vi "Auto2-CubeSwitch.vi"(5 "End By Time":timestamp, 7 "Start Time":timestamp, 11 "Game Data":string) -> (3 "Actual End Time":timestamp)   [LabVIEW 2017]
uses:
  AutoSubsystem/AutoInput.ctl
  AutoSubsystem/AutoSubroutine.lvclass
  DriveAutoData.ctl
  AutoSubsystem/AutoDrive/AutoDrive.lvclass
  AutoSubsystem/AutoOutput.ctl
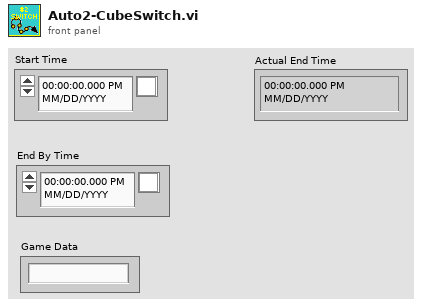
[diagram p1: front panel]
types:
  T1 = typedef "AutoSubroutine.lvclass/AutoInput.ctl" = cluster{"Start by (s)":dbl, "End by (s)":dbl, "Auto Start Time":timestamp, "Local Start":timestamp, "Okay To Start":bool, "End By Time":timestamp}
  T2 = typedef "AutoDrive.lvclass/DriveAutoData.ctl" = cluster{"LinearControlMethod":enum16{"Feedback", "Time"}, "Initial gyro angle":dbl}
  T3 = typedef "AutoSubroutine.lvclass/AutoOutput.ctl" = cluster{"Ended Safe?":bool, "True Start (s)":dbl, "True End (s)":dbl}
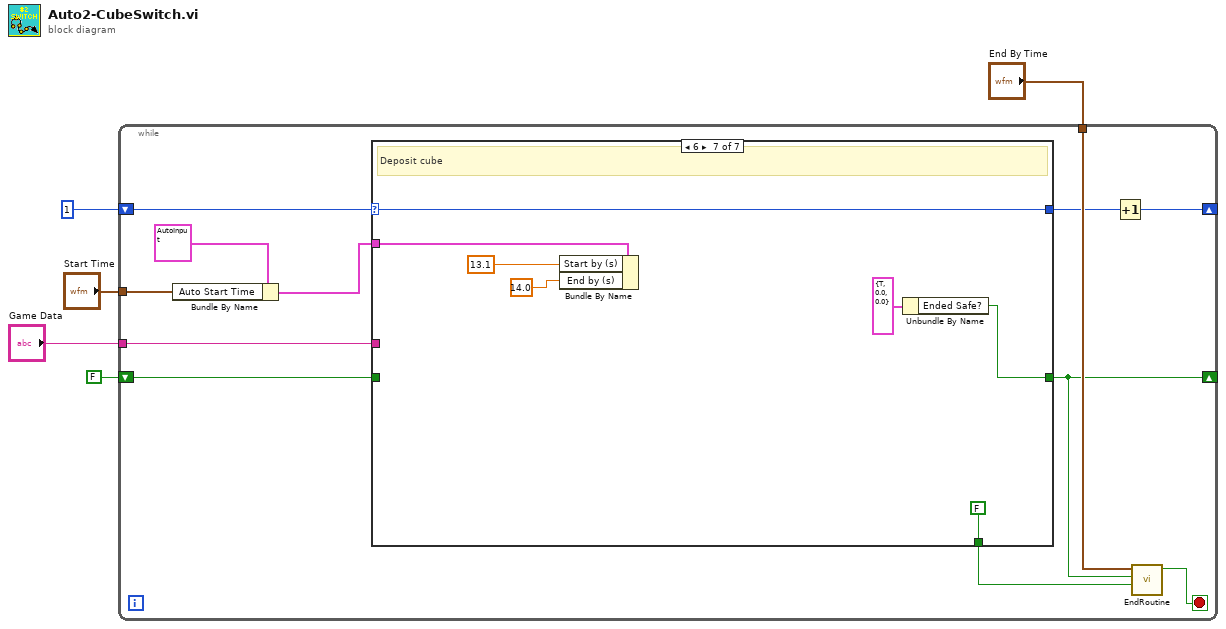
[diagram p0: block diagram]
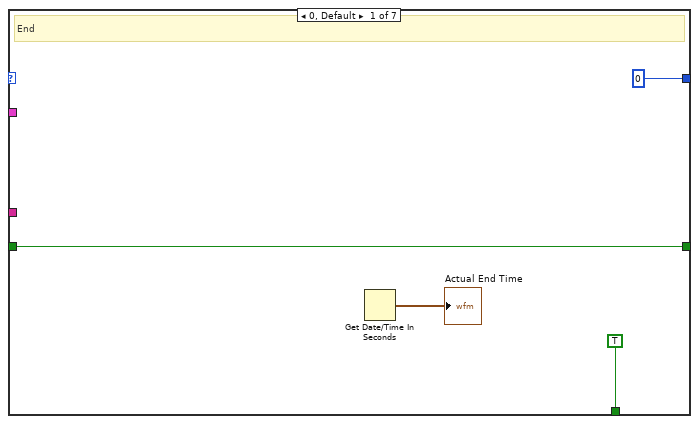
[diagram p2: hidden frame]
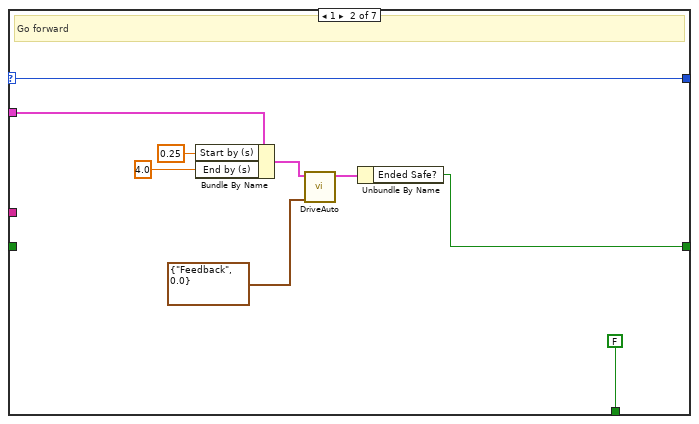
[diagram p3: hidden frame]
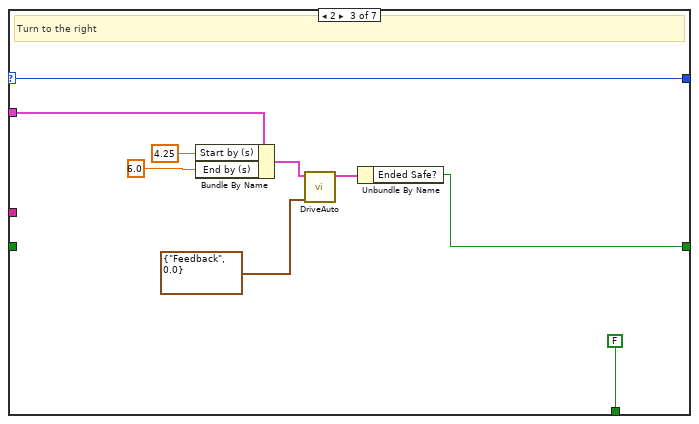
[diagram p4: hidden frame]
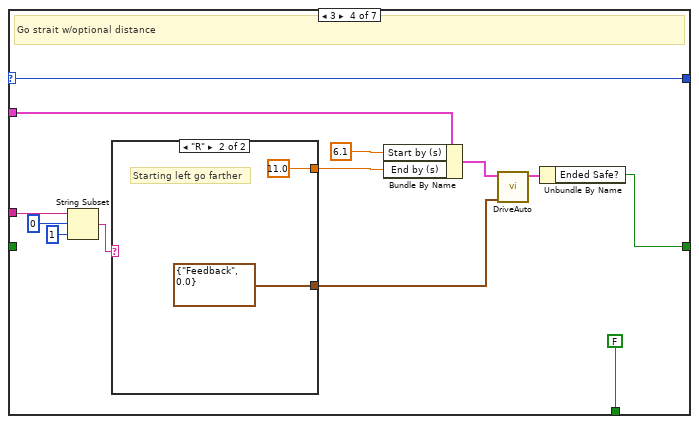
[diagram p5: hidden frame]
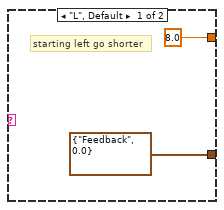
[diagram p6: hidden frame]
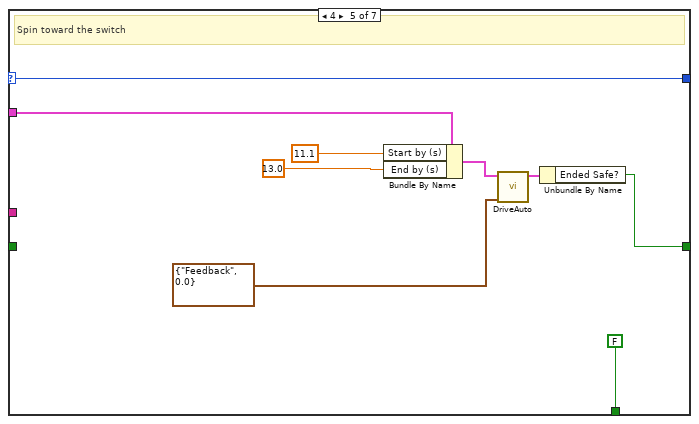
[diagram p7: hidden frame]
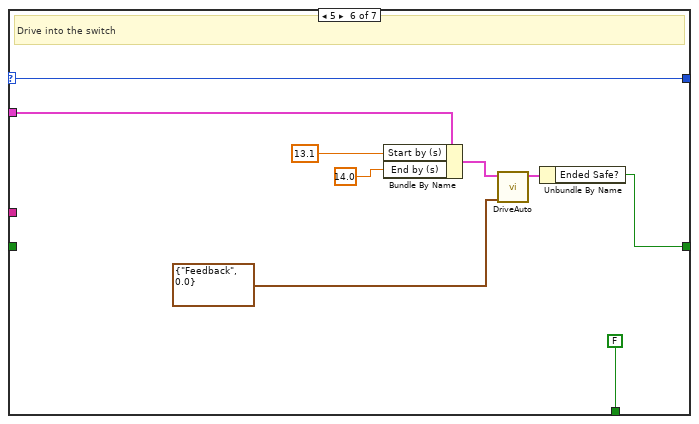
[diagram p8: hidden frame]
diagram:
  n1 = while {
    tunnel: "Start Time" -> [w9]
    tunnel: "End By Time" -> [w17]
    shift-right: [w6] -> _
    shift-left: 1 -> [w16]
    shift-right: [w12] -> _
    shift-left: FALSE ("Ended Safe?") -> [w13]
    tunnel: "Game Data" -> [w10]
    stop <- w14 stop-if-true
    n2 = Bundle By Name(cluster=T1 {"Start by (s)"=1.0, "End by (s)"=4.0, "Auto Start Time"=timestamp(0 s since 1904-01-01), "Local Start"=timestamp(0 s since 1904-01-01), "Okay To Start"=FALSE, "End By Time"=timestamp(0 s since 1904-01-01)} ("GeneralAutoInput"), "Auto Start Time"=w9) -> (w7:T1)
    n3 = case shown="6" w16 {
      selector: w16 -> [_ w22 w31 w41 w57 w66 w79]
      tunnel: [0 w22 w31 w41 w57 w66 w79] -> w15
      tunnel: w7 -> [_ w29 w38 w51 w64 w73 w75]
      tunnel: [w21 w24 w33 w47 w59 w68 w81] -> w12
      tunnel: w13 -> [w21 _ _ _ _ _ _]
      tunnel: [TRUE ("Ended Safe?") FALSE ("Ended Safe?") FALSE ("Ended Safe?") FALSE ("Ended Safe?") FALSE ("Ended Safe?") FALSE ("Ended Safe?") FALSE ("Ended Safe?")] -> w11
      tunnel: w10 -> [_ _ _ w45 _ _ _]
      frame 0, Default {
        # "End"
        n4 = Get Date/Time In Seconds() -> (seconds since 1Jan1904=→"Actual End Time":timestamp)
      }
      frame 1 {
        # "Go forward"
        n5 = Bundle By Name(cluster=w29, "Start by (s)"=0.25, "End by (s)"=4.0) -> (w25:T1)
        n6 = call "DriveAuto.vi"("DriveAutoInput"=T2 {"LinearControlMethod"=enum."Feedback", "Initial gyro angle"=0.0}, "GeneralAutoInput"=w25) -> ("AutoGeneralOut"=w26:T3)  [unwired: 9 in]
        n7 = Unbundle By Name(w26) -> ("Ended Safe?"=w24:bool)
      }
      frame 2 {
        # "Turn to the right"
        n8 = Bundle By Name(cluster=w38, "Start by (s)"=4.25, "End by (s)"=6.0) -> (w34:T1)
        n9 = call "DriveAuto.vi"("DriveAutoInput"=T2 {"LinearControlMethod"=enum."Feedback", "Initial gyro angle"=0.0}, "GeneralAutoInput"=w34) -> ("AutoGeneralOut"=w35:T3)  [unwired: 9 in]
        n10 = Unbundle By Name(w35) -> ("Ended Safe?"=w33:bool)
      }
      frame 3 {
        # "Go strait w/optional distance"
        n11 = String Subset(string=w45, offset (0)=0, length (rest)=1 ("length (rest)")) -> (substring=w42:string)
        n12 = case shown="\"R\"" w42 {
          tunnel: [T2 {"LinearControlMethod"=enum."Feedback", "Initial gyro angle"=0.0} ("DriveAutoInput") T2 {"LinearControlMethod"=enum."Feedback", "Initial gyro angle"=0.0} ("DriveAutoInput")] -> w52
          tunnel: [8.0 ("End by (s)") 11.0 ("End by (s)")] -> w50
          frame "L", Default {
            # "starting left go shorter"
          }
          frame "R" {
            # "Starting left go farther"
          }
        }
        n13 = Bundle By Name(cluster=w51, "Start by (s)"=6.1, "End by (s)"=w50) -> (w48:T1)
        n14 = call "DriveAuto.vi"("DriveAutoInput"=w52, "GeneralAutoInput"=w48) -> ("AutoGeneralOut"=w49:T3)  [unwired: 9 in]
        n15 = Unbundle By Name(w49) -> ("Ended Safe?"=w47:bool)
      }
      frame 4 {
        # "Spin toward the switch"
        n16 = Bundle By Name(cluster=w64, "Start by (s)"=11.1, "End by (s)"=13.0) -> (w60:T1)
        n17 = call "DriveAuto.vi"("DriveAutoInput"=T2 {"LinearControlMethod"=enum."Feedback", "Initial gyro angle"=0.0}, "GeneralAutoInput"=w60) -> ("AutoGeneralOut"=w61:T3)  [unwired: 9 in]
        n18 = Unbundle By Name(w61) -> ("Ended Safe?"=w59:bool)
      }
      frame 5 {
        # "Drive into the switch"
        n19 = Bundle By Name(cluster=w73, "Start by (s)"=13.1, "End by (s)"=14.0) -> (w69:T1)
        n20 = call "DriveAuto.vi"("DriveAutoInput"=T2 {"LinearControlMethod"=enum."Feedback", "Initial gyro angle"=0.0}, "GeneralAutoInput"=w69) -> ("AutoGeneralOut"=w70:T3)  [unwired: 9 in]
        n21 = Unbundle By Name(w70) -> ("Ended Safe?"=w68:bool)
      }
      frame 6 {
        # "Deposit cube"
        n22 = Bundle By Name(cluster=w75, "Start by (s)"=13.1, "End by (s)"=14.0) -> ()  [unwired: 1 out]
        n23 = Unbundle By Name(T3 {"Ended Safe?"=TRUE, "True Start (s)"=0.0, "True End (s)"=0.0} ("input cluster")) -> ("Ended Safe?"=w81:bool)
      }
    }
    n24 = Increment(x=w15) -> (x+1=w6:i32)
    n25 = call "EndRoutine.vi"("End?"=w11, "Ended Safe?"=w12, "End Time"=w17) -> ("Stop?"=w14:bool)  [unwired: 8 in]
  }
